vi "Teleop.vi"(10 "Match Info":T1={"Autonomous Elapsed Seconds"=0.0, "TeleOp Elapsed Seconds"=0.0, "Disabled Elapsed Seconds"=0.0, "Visited Autonomous"=FALSE, "Visited TeleOp"=FALSE, "Visited Disabled"=FALSE, "Autonomous Settings"={"Autonomous Style"=enum."Independent", "VI Refnum"=refnum}}, 11 "Call Context":T2) -> ()   [LabVIEW 2018]
doc: "This VI is called for each enabled TeleOp packet received from the DS. It is typically used to read from joysticks and other inputs and update I/O or setpoints for timed control loops. It should complete and return within 20 milliseconds or risk missing DS packets."
uses:
  <vilib>/Rock Robotics/WPI/DriverStation/WPI_DriverStationDerivedRobotMode.ctl
  <vilib>/Rock Robotics/WPI/DriverStation/WPI_DriverStationMatch Info.ctl
  <vilib>/Rock Robotics/WPI/Solenoid/WPI_SolenoidValue.ctl
  Framework/Robot Global Data.vi
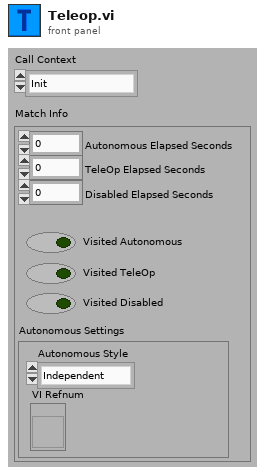
[diagram p1: front panel]
types:
  T1 = typedef "WPI_DriverStationMatch Info.ctl" = cluster{"Autonomous Elapsed Seconds":dbl, "TeleOp Elapsed Seconds":dbl, "Disabled Elapsed Seconds":dbl, "Visited Autonomous":bool, "Visited TeleOp":bool, "Visited Disabled":bool, "Autonomous Settings":cluster{"Autonomous Style":enum16{"Iterative", "Independent"}, "VI Refnum":refnum<vi>}}
  T2 = typedef "WPI_DriverStationDerivedRobotMode.ctl" = enum16{"Init", "Execute", "Stop"}
  T3 = typedef "Command Status Info.ctl" = cluster{"Name":string, "Status":T4, "notifier out":T5}
  T4 = typedef "Completion Status.ctl" = enum16{"Successful", "Aborted", "Incomplete"}
  T5 = typedef "Completion Notifier.ctl" = refnum<notifier>
  T6 = typedef "WPI_SolenoidValue.ctl" = enum16{"Off", "On", "Forward", "Reverse"}
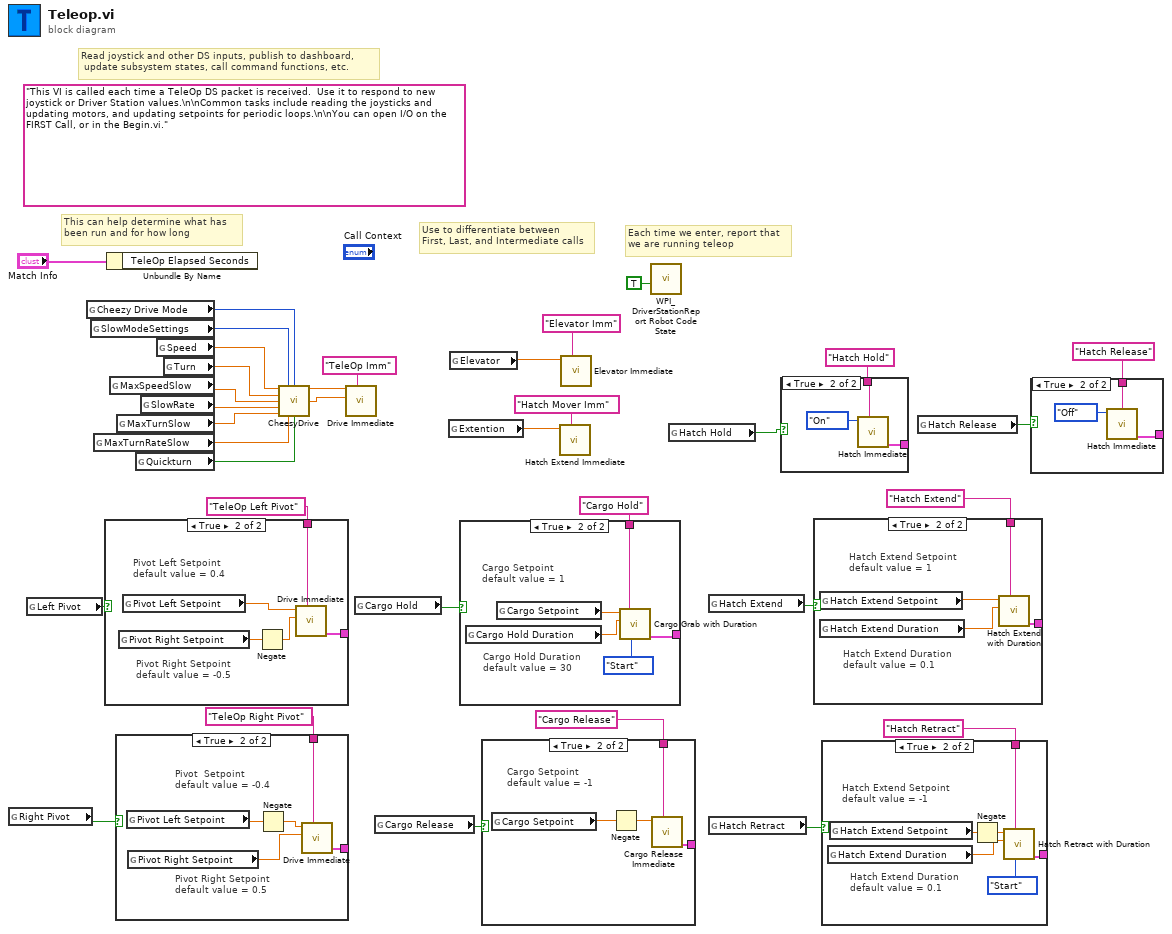
[diagram p0: block diagram]
diagram:
  (unwired) "This VI is called each time a TeleOp DS packet is received.  Use it to respond to new joystick or Driver Station values.\n\nCommon tasks include reading the joysticks and updating motors, and updating setpoints for periodic loops.\n\nYou can open I/O on the FIRST Call, or in the Begin.vi."
  # "Read joystick and other DS inputs, publish to dashboard,\n update subsystem states, call command functions, etc."
  # "Each time we enter, report that\nwe are running teleop"
  # "Use to differentiate between\nFirst, Last, and Intermediate calls"
  # "This can help determine what has\nbeen run and for how long"
  n1 = global read "Robot Global Data.vi" "Right Pivot"() -> (w30:bool)
  n2 = global read "Robot Global Data.vi" "Left Pivot"() -> (w29:bool)
  n3 = global read "Robot Global Data.vi" "Cheezy Drive Mode"() -> (w11:u32)
  n4 = global read "Robot Global Data.vi" "SlowModeSettings"() -> (w1:i32)
  n5 = global read "Robot Global Data.vi" "MaxTurnRateSlow"() -> (w3:dbl)
  n6 = case shown="True" w29 {
    tunnel: [_ w39] -> _
    tunnel: "TeleOp Left Pivot" ("Description") -> [_ w38]
    frame False {
    }
    frame True {
      # "Pivot Right Setpoint\ndefault value = -0.5"
      # "Pivot Left Setpoint\ndefault value = 0.4"
      n7 = global read "Robot Global Data.vi" "Pivot Right Setpoint"() -> (w36:dbl)
      n8 = global read "Robot Global Data.vi" "Pivot Left Setpoint"() -> (w37:dbl)
      n9 = Negate(x=w36) -> (-x=w35:dbl)
      n10 = call "Drive Immediate.vi"("Description"=w38, "Right Setpoint"=w35, "Left Setpoint"=w37) -> ("Command Info Out"=w39:T3)  [unwired: 8 in]
    }
  }
  n11 = Unbundle By Name("Match Info") -> ()  [unwired: 1 out]
  n12 = global read "Robot Global Data.vi" "MaxSpeedSlow"() -> (w6:dbl)
  n13 = case shown="True" w30 {
    tunnel: [_ w44] -> _
    tunnel: "TeleOp Right Pivot" ("Description") -> [_ w43]
    frame False {
    }
    frame True {
      # "Pivot Right Setpoint\ndefault value = 0.5"
      # "Pivot  Setpoint\ndefault value = -0.4"
      n14 = global read "Robot Global Data.vi" "Pivot Left Setpoint"() -> (w41:dbl)
      n15 = global read "Robot Global Data.vi" "Pivot Right Setpoint"() -> (w42:dbl)
      n16 = Negate(x=w41) -> (-x=w40:dbl)
      n17 = call "Drive Immediate.vi"("Description"=w43, "Right Setpoint"=w42, "Left Setpoint"=w40) -> ("Command Info Out"=w44:T3)  [unwired: 8 in]
    }
  }
  n18 = global read "Robot Global Data.vi" "MaxTurnSlow"() -> (w4:dbl)
  n19 = global read "Robot Global Data.vi" "Quickturn"() -> (w2:bool)
  n20 = global read "Robot Global Data.vi" "SlowRate"() -> (w5:dbl)
  n21 = global read "Robot Global Data.vi" "Speed"() -> (w8:dbl)
  n22 = global read "Robot Global Data.vi" "Turn"() -> (w7:dbl)
  n23 = call "CheesyDrive.vi"("Throttle"=w8, "SlowModeSettings"=w1, "SlowMode"=w11, "Wheel"=w7, "MaxSpeedSlow"=w6, "SlowRate"=w5, "MaxTurnSlow"=w4, "MaxTurnRateSlow"=w3, "Quickturn"=w2) -> ("Left PWM"=w10:dbl, "Right PWM"=w9:dbl)  [unwired: 5 in]
  n24 = call "Drive Immediate.vi"("Description"="TeleOp Imm", "Right Setpoint"=w9, "Left Setpoint"=w10) -> ()  [unwired: 8 in, 1 out]
  n25 = global read "Robot Global Data.vi" "Cargo Hold"() -> (w24:bool)
  n26 = global read "Robot Global Data.vi" "Cargo Release"() -> (w23:bool)
  n27 = global read "Robot Global Data.vi" "Extention"() -> (w14:dbl)
  n28 = global read "Robot Global Data.vi" "Elevator"() -> (w28:dbl)
  n29 = case shown="True" w24 {
    tunnel: [_ w49] -> _
    tunnel: "Cargo Hold" ("Description") -> [_ w48]
    frame False {
    }
    frame True {
      # "Cargo Hold Duration\ndefault value = 30"
      # "Cargo Setpoint\ndefault value = 1"
      n30 = global read "Robot Global Data.vi" "Cargo Hold Duration"() -> (w45:dbl)
      n31 = global read "Robot Global Data.vi" "Cargo Setpoint"() -> (w47:dbl)
      n32 = call "Cargo Grab with Duration.vi"("Synchronization"=enum16{"Start", "Wait"}."Start", "Description"=w48, "Duration (s)"=w45, "Setpoint"=w47) -> ("Command Info Out"=w49:T3)  [unwired: 7 in]
    }
  }
  n33 = case shown="True" w23 {
    tunnel: [_ w53] -> _
    tunnel: "Cargo Release" ("Description") -> [_ w52]
    frame False {
    }
    frame True {
      # "Cargo Setpoint\ndefault value = -1"
      n34 = global read "Robot Global Data.vi" "Cargo Setpoint"() -> (w51:dbl)
      n35 = Negate(x=w51) -> (-x=w50:dbl)
      n36 = call "Cargo Release Immediate.vi"("Description"=w52, "Setpoint"=w50) -> ("Command Info Out"=w53:T3)  [unwired: 9 in]
    }
  }
  n37 = call "Hatch Extend Immediate.vi"("Description"="Hatch Mover Imm", "Setpoint"=w14) -> ()  [unwired: 9 in, 1 out]
  n38 = call "Elevator Immediate.vi"("Description"="Elevator Imm", "Setpoint"=w28) -> ()  [unwired: 9 in, 1 out]
  n39 = call <vilib>:"WPI_DriverStationReport Robot Code State.vi"("TeleOp"=TRUE ("Autonomous")) -> ()  [unwired: 10 in, 1 out]
  n40 = global read "Robot Global Data.vi" "Hatch Hold"() -> (w19:bool)
  n41 = global read "Robot Global Data.vi" "Hatch Extend"() -> (w18:bool)
  n42 = global read "Robot Global Data.vi" "Hatch Retract"() -> (w17:bool)
  n43 = case shown="True" w19 {
    tunnel: "Hatch Hold" ("Description") -> [_ w56]
    tunnel: [_ w55] -> _
    frame False {
    }
    frame True {
      n44 = call "Hatch Immediate.vi"("Description"=w56, "Relay Value"=WPI_SolenoidValue."On" ("Hatch Action")) -> ("Command Info Out"=w55:T3)  [unwired: 9 in]
    }
  }
  n45 = case shown="True" w18 {
    tunnel: [_ w60] -> _
    tunnel: "Hatch Extend" ("Description") -> [_ w59]
    frame False {
    }
    frame True {
      # "Hatch Extend Duration\ndefault value = 0.1"
      # "Hatch Extend Setpoint\ndefault value = 1"
      n46 = global read "Robot Global Data.vi" "Hatch Extend Setpoint"() -> (w58:dbl)
      n47 = global read "Robot Global Data.vi" "Hatch Extend Duration"() -> (w57:dbl)
      n48 = call "Hatch Extend with Duration.vi"("Description"=w59, "Duration (s)"=w57, "Setpoint"=w58) -> ("Command Info Out"=w60:T3)  [unwired: 8 in]
    }
  }
  n49 = case shown="True" w17 {
    tunnel: [_ w66] -> _
    tunnel: "Hatch Retract" ("Description") -> [_ w65]
    frame False {
    }
    frame True {
      # "Hatch Extend Setpoint\ndefault value = -1"
      # "Hatch Extend Duration\ndefault value = 0.1"
      n50 = global read "Robot Global Data.vi" "Hatch Extend Duration"() -> (w62:dbl)
      n51 = global read "Robot Global Data.vi" "Hatch Extend Setpoint"() -> (w64:dbl)
      n52 = Negate(x=w64) -> (-x=w61:dbl)
      n53 = call "Hatch Retract with Duration.vi"("Synchronization"=enum16{"Start", "Wait"}."Start", "Description"=w65, "Duration (s)"=w62, "Setpoint"=w61) -> ("Command Info Out"=w66:T3)  [unwired: 7 in]
    }
  }
  n54 = global read "Robot Global Data.vi" "Hatch Release"() -> (w20:bool)
  n55 = case shown="True" w20 {
    tunnel: "Hatch Release" ("Description") -> [_ w69]
    tunnel: [_ w68] -> _
    frame False {
    }
    frame True {
      n56 = call "Hatch Immediate.vi"("Description"=w69, "Relay Value"=WPI_SolenoidValue."Off" ("Hatch Action")) -> ("Command Info Out"=w68:T3)  [unwired: 9 in]
    }
  }
